vi "Copy Pixmap to Image (Greyscale Flatten Mask).vi"(7 "Value (Default: 0)":u8, 8 "error in (no error)":errorcluster, 10 "Greyscale Image Destination":T2, 11 "Pixmap Image Data":T1) -> (0 "error out":errorcluster, 3 "Greyscale Image Destination (duplicate)":T2)   [LabVIEW 2020, in "g_ar_toolkit.image.lvlib"]
uses:
  g_ar_toolkit.image.lvlib
  Greyscale Image.ctl
  <vilib>/picture/picture.llb/imagedata.ctl
  f0818824-bd55-4656-87f2-fcc208e7cf24.vi
  FixPixmap.vi
  Default8bitColourMap.vi
  <vilib>/Utility/error.llb/Error Cluster From Error Code.vi
  g_ar_toolkit.common/Module Path.vi
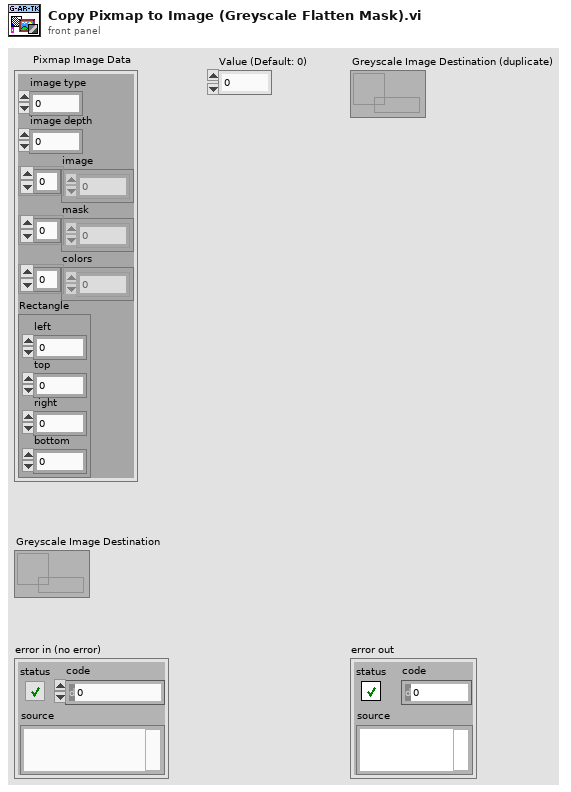
[diagram p1: front panel]
types:
  T1 = typedef "imagedata.ctl" = cluster{"image type":i32, "image depth":i32, "image":u8[], "mask":u8[], "colors":u32[], "Rectangle":cluster{"left":i16, "top":i16, "right":i16, "bottom":i16}}
  T2 = typedef "g_ar_toolkit.image.lvlib/Greyscale Image.ctl" = refnum<data-value>
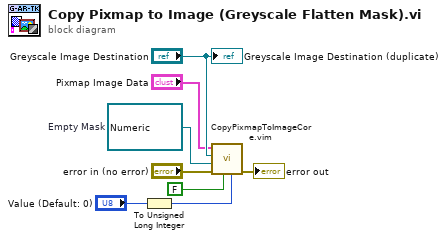
[diagram p0: block diagram]
diagram:
  w3 = refnum<data-value> refnum  # Empty Mask
  n1 = To Unsigned Long Integer(number="Value (Default: 0)") -> (unsigned 32bit integer=w1:u32)
  n2 = call "CopyPixmapToImageCore.vim"("Background Value"=w1, "Has Mask"=FALSE, "error in (no error)"="error in (no error)", "Mask Image"=w3, "Source Image"="Greyscale Image Destination", "image data"="Pixmap Image Data") -> ("error out"=→"error out":errorcluster)  [unwired: 5 in]
  "Greyscale Image Destination (duplicate)" <- "Greyscale Image Destination"
